vi "Y Goal Marker.vi"(0 "dest_y_kick":dbl, 1 "Touch":bool, 5 "ball x":dbl, 9 "ball y":dbl, 11 "goal width":dbl, 12 "goal x":dbl) -> (4 "Goal or Not":bool, 6 "kick error":dbl)   [LabVIEW 2017]
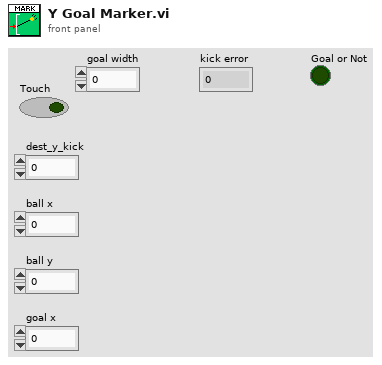
[diagram p1: front panel]
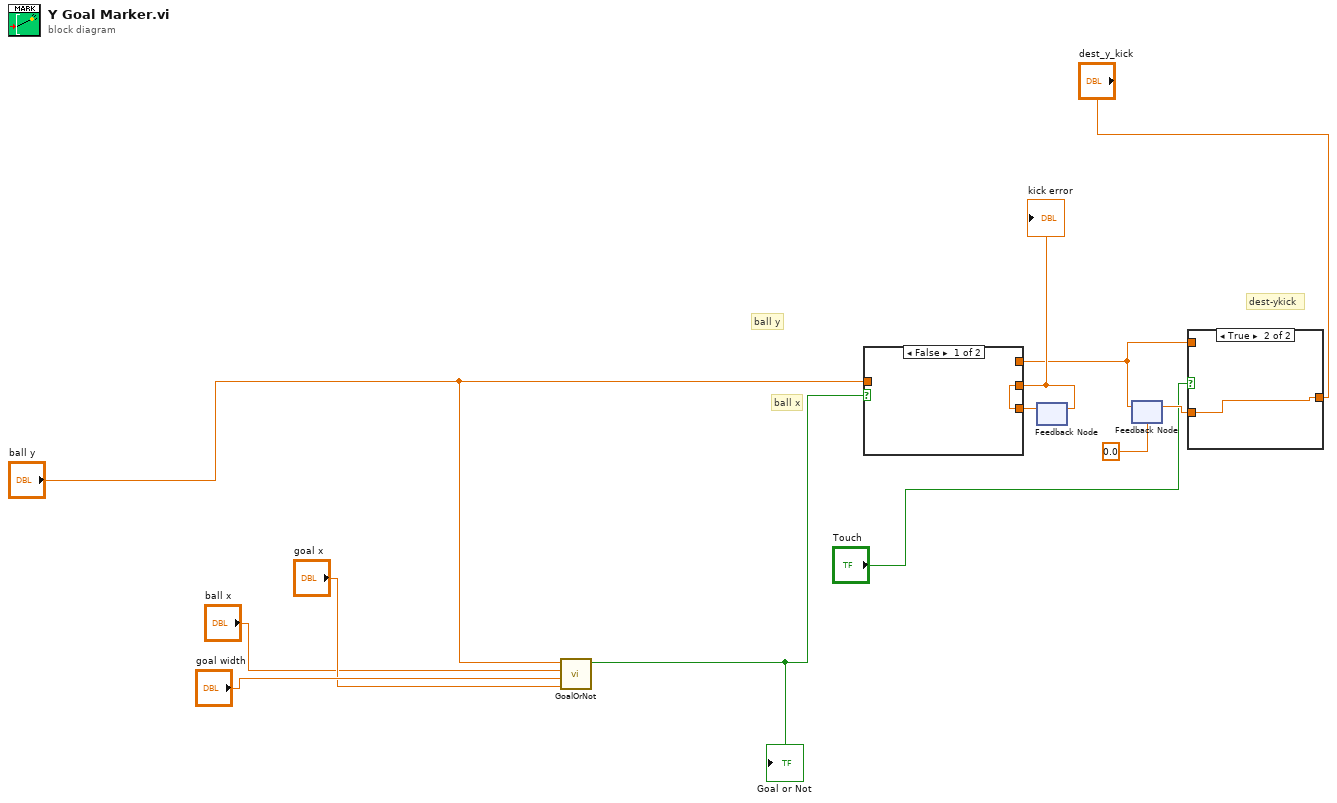
[diagram p0: block diagram]
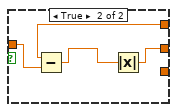
[diagram p2: hidden frame]
diagram:
  # "dest-ykick"
  # "ball y"
  # "ball x"
  n1 = call "GoalOrNot.vi"("goal x"="goal x", "goal width"="goal width", "ball x"="ball x", "ball y"="ball y") -> ("Goal or Not"=w5:bool)  [unwired: 7 in]
  "Goal or Not" <- w5
  n2 = feedback #1() -> (w12:dbl)  [unwired: 1 in]
  n3 = feedback #2(0.0 ("dest_y")) -> (w10:dbl)
  n4 = case shown="False" w5 {
    tunnel: w10 -> [_ w17]
    tunnel: "ball y" -> [_ w14]
    tunnel: [w13 w15] -> w11
    tunnel: w12 -> [w13 _]
    frame False {
    }
    frame True {
      n5 = Subtract(x=w17, y=w14) -> (x-y=w16:dbl)
      n6 = Absolute Value(x=w16) -> (abs(x)=w15:dbl)
    }
  }
  "kick error" <- w11
  n7 = feedback-in #1(w11) -> ()
  n8 = case shown="True" "Touch" {
    tunnel: "dest_y_kick" -> [_ w19]
    tunnel: [w18 w19] -> w8
    tunnel: w10 -> [w18 _]
    frame False {
    }
    frame True {
    }
  }
  n9 = feedback-in #2(w8) -> ()
